vi "Blocker.vi"(7 "block?":bool, 8 "Error in":errorcluster) -> (0 "Error Out":errorcluster)   [LabVIEW 2018]
uses:
  type defines/Pause action.ctl
  Controls/FGV Actions.ctl
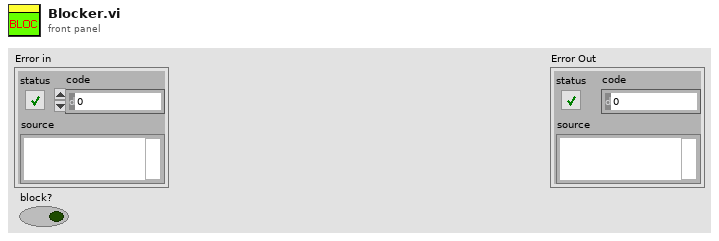
[diagram p1: front panel]
types:
  T1 = typedef "FGV Actions.ctl" = enum16{"Init", "Set", "Get", "Clear"}
  T2 = typedef "Pause action.ctl" = enum16{"Init", "get", "set"}
  T3 = typedef "System Parameters.ctl" = cluster{"Optical Parameters":T4, "Vibratome":T5, "Table Stages":T7, "Imaging Parameter":T10, "Galvo HW Parameters":cluster{"Analog Out Channel":tag, "Min Voltage":dbl, "Max Voltage":dbl, "Pixel Clock Source":tag, "Sample Rate":dbl, "Line Clock Out Ch":tag, "2P ready check":tag}, "Alazar parameters":T12, "Mosaic Paramter":cluster{"X Axis":cluster{"Start [mm]":dbl, "Steps [pts]":dbl, "End [mm]":dbl}, "Y Axis":cluster{"Start [mm]":dbl, "Steps [pts]":dbl, "End [mm]":dbl}, "Scan Pattern":enum16{"Uni-directional", "Bi-Directional", "Spiral Out", "Spiral In"}, "Overlap Options":cluster{"Overlap Type":enum16{"No Overlap", "X Only", "Y Only", "X and Y"}, "Percent Overlap":u8, "Justify":enum16{"Start", "Center", "End"}}}, "Manual Controls":T19, "Z stage setting":T22, "Attenuator":T23}
  T4 = typedef "Optical Parameters.ctl" = cluster{"Obj. Focal Length [mm]":dbl, "Scan Lens EFL[mm]":dbl, "Tube Lens EFL[mm]":dbl, "Galvo V Range (+/-)":dbl, "Galvo Max Half Angle [Deg]":dbl, "Max Galvo Range[%]":dbl}
  T5 = typedef "Vibratome Parameters.ctl" = cluster{"Pre Cut Dwell [s]":dbl, "Blade Frequency [RPM]":u16, "Slice Speed [mm/s]":dbl, "Post Cut Dwell [s]":dbl, "Ramp Time [s]":dbl, "Start X [mm]":dbl, "Start Y [mm]":dbl, "Slice Length [mm]":dbl, "Slice Axis":enum16{"X Axis", "Y Axis", "Z Axis"}, "Controller VISA Ref":refnum<visa-resource-name>, "Blade Frequency [Hz]":u16, "Analog Out Channel":tag, "Pixel Clock Source":tag, "Vib version":T6}
  T6 = typedef "vibratome.ctl" = enum16{"Vibratome1", "Vibratome3"}
  T7 = typedef "Translation Stage Parameters.ctl" = cluster{"X Stage":T8, "Y Stage":T8, "Z Stage":T8, "Attenuator":T8}
  T8 = typedef "Translation Stage Cluster.ctl" = cluster{"Position":dbl, "Is.Enabled?":bool, "Is.Connected?":bool, "Device SN":string, "AccelerationMaximum":dbl, "VelocityMaximum":dbl, "Acceleration":dbl, "Velocity":dbl, "waitTimeout (ms)":i32, "Model":T9, "Is.Homed?":bool, "MOVE":bool}
  T9 = typedef "Translation Stage Types.ctl" = enum16{"None", "Thorlabs LTS", "Thorlabs MLJ"}
  T10 = typedef "Imaging Parameters.ctl" = cluster{"Raster Scan Direction":T11, "Pixel Dwell Time [Clock Cycles]":u16, "Flyback Time [Clock Cycles]":u16, "XY Center [um]":cluster{"X":dbl, "Y":dbl}, "Pixel Step Size [um] X":dbl, "XY Image Size":enum16{"32 x 32", "64 x 64", "128 x 128", "256 x 256", "512 x 512", "1024 x 1024", "2048 x 2048"}, "Custom":bool, "Custom Size":cluster{"X":u16, "Y":u16}, "Line Averages":u8, "Pixel Step Size [um] Y":dbl}
  T11 = typedef "Scan Direction.ctl" = enum16{"Uni Directional", "Bi Directional", "None"}
  T12 = typedef "Alazar parameters.ctl" = cluster{"Trigger Settings":cluster{"General Trigger Settings":T13, "Trigger Engine 1":T14, "Trigger Engine 2":T14}, "Device ID":T15, "Ch A Input Control":T16, "Ch B Input Control":T16, "Acq Settings":T17, "Capture Clock":T18}
  T13 = typedef "General Trigger Settings.ctl" = cluster{"Trigger Operation":u32, "Coupling ID":u32, "Range ID":u32, "Delay":u32, "Timeout Ticks":u32, "Mode":u32, "Parameter":u32}
  T14 = typedef "Trigger Engine Controls.ctl" = cluster{"Trigger Engine":u32, "Source":u32, "Slope":u32, "Level":u32}
  T15 = typedef "Alazar Device ID.ctl" = cluster{"System ID":u32, "Board ID":u32}
  T16 = typedef "Channel Input Controls.ctl" = cluster{"Channel":u8, "Coupling":u32, "Range":u32, "Impedance":u32}
  T17 = typedef "Alazar Acquisition Settings.ctl" = cluster{"Record Length":u32, "Offset":u32, "Records Per Buffer":u32, "Records Count (Records/Acq)":u32, "Window Type":u32, "Footer":u32, "Samples per record":u32, "Output Format":u32}
  T18 = typedef "Clock Controls.ctl" = cluster{"Sample Rate":u32, "Decimation":u32, "Source":u32, "Edge":u32}
  T19 = typedef "Manual Controls.ctl" = cluster{"Data Path":path, "Save parameters":T20, "Center Galvos":bool, "Acquisition mode":T21, "PSOCT Channel":u32, "Save data?":bool, "AIP rotation angle":dbl, "Pause acquisition?":bool, "Outgoing Mail Server (SMTP)":string, "Email":string, "Password":string, "Carrier 1":enum16{"T-Mobile", "AT&T", "Verizon", "Sprint"}, "phone number 1":string, "Subject":string, "Message":string, "Carrier 2":enum16{"T-Mobile", "AT&T", "Verizon", "Sprint"}, "phone number 2":string, "Check boundary?":bool, "Threshold":sgl, "ret downsample?":bool}
  T20 = typedef "FFT parameters.ctl" = cluster{"start pixel":i32, "#pixels to save":i32}
  T21 = typedef "FFT mode.ctl" = enum16{"ThorOCT B line", "ThorOCT Spectral", "ThorOCT FFT", "Alazar B line", "Alazar FFT", "GPU FFT", "Alazar Spectral", "Simulation", "auto adjust focus", "Save all"}
  T22 = typedef "Vibratome Param.ctl" = cluster{"first cut height(mm)":dbl, "slice thickness[um]":dbl[], "#repetitions":u16, "image thickness(um)":dbl[], "#cycles per repetition":u16, "First image height(mm)":dbl, "Block?":bool[], "Z0":dbl, "fixed Z0?":bool}
  T23 = typedef "attenuator.ctl" = cluster{"Power after Objective (recalibrate every 6 month)":dbl[]}
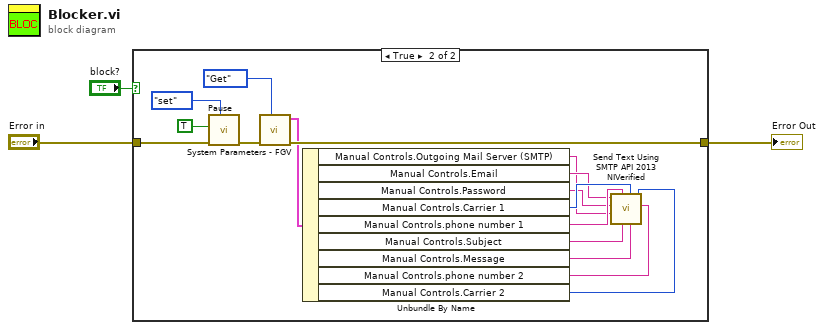
[diagram p0: block diagram]
diagram:
  n1 = case shown="True" "block?" {
    tunnel: "Error in" -> [w4 w18]
    tunnel: [w4 w16] -> w2
    frame False {
    }
    frame True {
      n2 = call "Pause.vi"("action"=Pause_action."set", "error in"=w18, "Pause!"=TRUE) -> ("error out"=w17:errorcluster)  [unwired: 7 in, 1 out]
      n3 = call "System Parameters - FGV.vi"("Actions"=FGV_Actions."Get", "Error In"=w17) -> ("Error Out"=w16:errorcluster, "System Parameters [Out]"=w14:T3)  [unwired: 8 in]
      n4 = Unbundle By Name(w14) -> ("Manual Controls.Outgoing Mail Server (SMTP)"=w7:string, "Manual Controls.Email"=w11:string, "Manual Controls.Password"=w10:string, "Manual Controls.Carrier 1"=w13:enum16{"T-Mobile", "AT&T", "Verizon", "Sprint"}, "Manual Controls.phone number 1"=w12:string, "Manual Controls.Subject"=w9:string, "Manual Controls.Message"=w8:string, "Manual Controls.phone number 2"=w6:string, "Manual Controls.Carrier 2"=w5:enum16{"T-Mobile", "AT&T", "Verizon", "Sprint"})
      n5 = call "Send Text Using SMTP API 2013 NIVerified.vi"("phone number 2"=w6, "Carrier 2"=w5, "Body"=w8, "Carrier 1"=w13, "Subject"=w9, "phone number 1"=w12, "Outgoing Mail Server (SMTP)"=w7, "Password"=w10, "Email"=w11) -> ()  [unwired: 3 in]
    }
  }
  "Error Out" <- w2
